vi "Get Result.vi"(8 "error in (no error)":errorcluster, 11 "AverageCollector2D in":refnum<class "AverageCollector2D.lvclass">) -> (0 "error out":errorcluster, 2 "Collected Result out":refnum<class "AbstractData.lvclass">, 3 "AverageCollector2D out":refnum<class "AverageCollector2D.lvclass">)   [LabVIEW 2014, in "AverageCollector2D.lvclass"]
uses:
  AverageCollector2D.lvclass
  Framework/Model/Data/AbstractData/AbstractData.lvclass
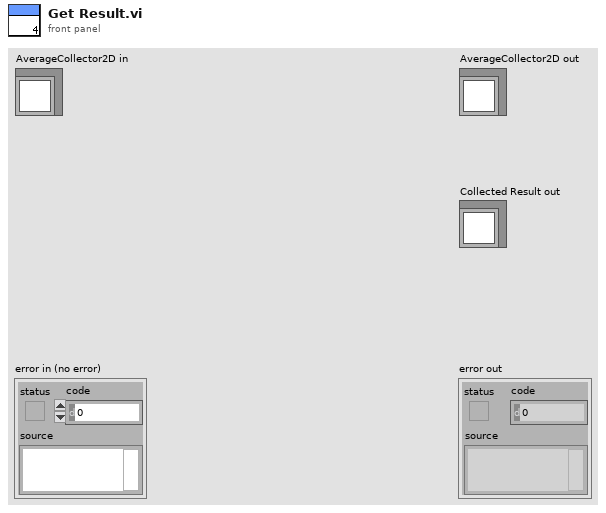
[diagram p1: front panel]
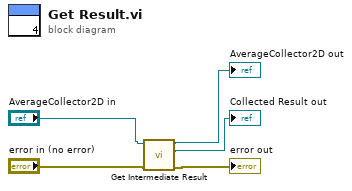
[diagram p0: block diagram]
diagram:
  n1 = call-dynamic "Get Intermediate Result.vi"("error in (no error)"="error in (no error)", "AverageCollector2D in"="AverageCollector2D in") -> ("error out"=→"error out":errorcluster, "AbstractData.lvclass"=→"Collected Result out":refnum<class "AbstractData.lvclass">, "AverageCollector2D out"=→"AverageCollector2D out":refnum<class "AverageCollector2D.lvclass">)  [unwired: 7 in]
